vi "tm_setcooling.vi"(8 "error in (no error)":errorcluster, 10 "Mode":bool, 11 "Handle in":u32) -> (0 "error out":errorcluster, 3 "Handle out":u32)   [LabVIEW 2012]
uses:
  tmcamcon.dll
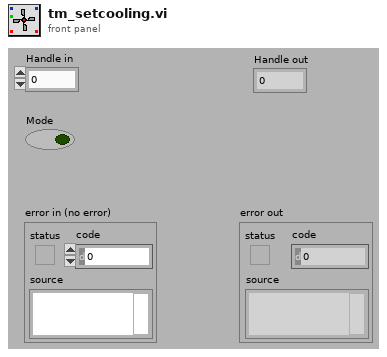
[diagram p1: front panel]
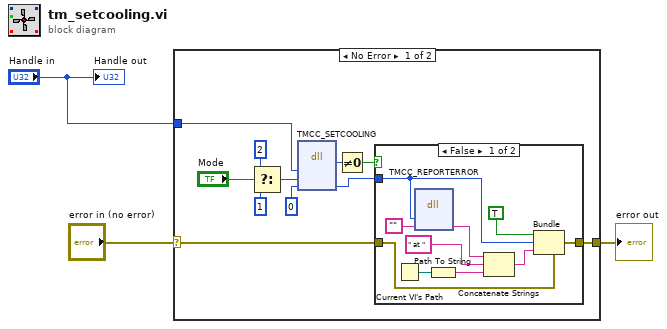
[diagram p0: block diagram]
diagram:
  n1 = case shown="No Error" "error in (no error)" {
    selector: "error in (no error)" -> [w8 w26]
    tunnel: [w5 w26] -> w2
    tunnel: "Handle in" -> [w4 _]
    frame No Error {
      n2 = Select(t=2, s="Mode", f=1) -> (s? t:f=w10:i32)
      n3 = dll-call lib="tmcamcon.dll" fn="TMCC_SETCOOLING"("HDCAM"=w4, "mode"=w10, "Erval"=0) -> ("return type"=w14:u32, "Erval"=w7:i32)  [unwired: 5 in, 2 out]
      n4 = Not Equal To 0?(x=w14) -> (x != 0?=w6:bool)
      n5 = case shown="False" w6 {
        tunnel: w8 -> [w24 w25]
        tunnel: [w23 w25] -> w5
        tunnel: w7 -> [w17 _]
        frame False {
          n6 = Current VI's Path() -> (path=w22:path)
          n7 = dll-call lib="tmcamcon.dll" fn="TMCC_REPORTERROR"("error"=w17, "buf"="") -> ("buf"=w16:string)  [unwired: 5 in, 2 out]
          n8 = Path To String(path=w22) -> (string=w18:string)
          n9 = Concatenate Strings(w16, " at ", w18) -> (w21:string)
          n10 = Bundle(cluster=w24, "status"=TRUE, "code"=w17, "source"=w21) -> (w23:errorcluster)
        }
        frame True {
        }
      }
    }
    frame Error {
    }
  }
  "error out" <- w2
  "Handle out" <- "Handle in"
